vi "InitCam3001.vi"(7 "error in (no error)":errorcluster, 8 "trigger_input":u16, 10 "IS_AREA":u16) -> (0 "error out":errorcluster)   [LabVIEW 2015, in "ESLSCDLL.lvlib"]
uses:
  ESLSCDLL.lvlib
  Globals.vi
  ESLSCDLL.dll
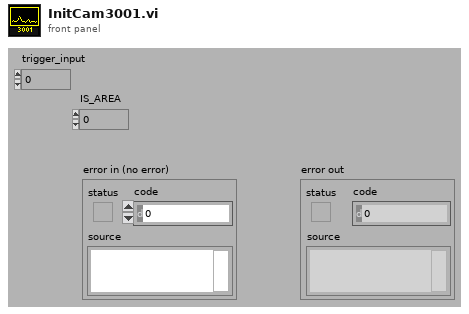
[diagram p1: front panel]
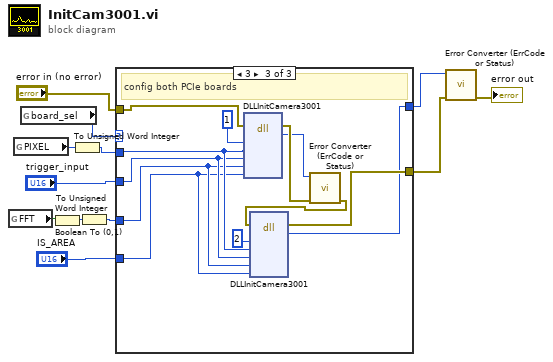
[diagram p0: block diagram]
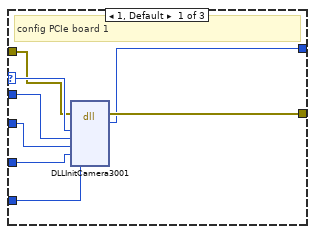
[diagram p2: hidden frame]
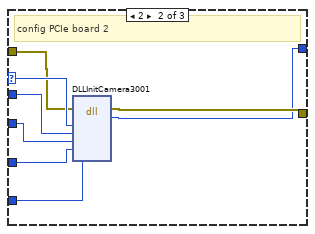
[diagram p3: hidden frame]
diagram:
  n1 = global read "Globals.vi" "FFT"() -> (w5:bool)
  n2 = global read "Globals.vi" "PIXEL"() -> (w2:u32)
  n3 = global read "Globals.vi" "board_sel"() -> (w6:u32)
  n4 = Boolean To (0,1)(Boolean=w5) -> (0, 1=w4:i16)
  n5 = To Unsigned Word Integer(number=w2) -> (unsigned 16bit integer=w1:u16)
  n6 = To Unsigned Word Integer(number=w4) -> (unsigned 16bit integer=w3:u16)
  n7 = case shown="3" w6 {
    selector: w6 -> [w20 w28 _]
    tunnel: w1 -> [w19 w27 w38]
    tunnel: "trigger_input" -> [w18 w26 w37]
    tunnel: w3 -> [w17 w25 w36]
    tunnel: "IS_AREA" -> [w16 w24 w35]
    tunnel: "error in (no error)" -> [w15 w23 w34]
    tunnel: [w14 w22 w30] -> w8
    tunnel: [w13 w21 w29] -> w7
    frame 1, Default {
      # "config PCIe board 1"
      n8 = dll-call lib="C:/Users/flori/Nextcloud/Dokumente/Stresing/Windows/lv64/board.vis/ESLSCDLL.dll" fn="DLLInitCamera3001" ("lwlscdll.dll:DLLWriteLongS0")(error in=w15, "drvno"=w20, "pixel"=w19, "trigger_input"=w18, "IS_FFT"=w17, "IS_AREA"=w16) -> (error out=w14:errorcluster, "es_status_codes"=w13:i32)  [unwired: 7 in, 1 out]
    }
    frame 2 {
      # "config PCIe board 2"
      n9 = dll-call lib="C:/Users/flori/Nextcloud/Dokumente/Stresing/Windows/lv64/board.vis/ESLSCDLL.dll" fn="DLLInitCamera3001" ("lwlscdll.dll:DLLWriteLongS0")(error in=w23, "drvno"=w28, "pixel"=w27, "trigger_input"=w26, "IS_FFT"=w25, "IS_AREA"=w24) -> (error out=w22:errorcluster, "es_status_codes"=w21:i32)  [unwired: 7 in, 1 out]
    }
    frame 3 {
      # "config both PCIe boards"
      n10 = dll-call lib="C:/Users/flori/Nextcloud/Dokumente/Stresing/Windows/lv64/board.vis/ESLSCDLL.dll" fn="DLLInitCamera3001" ("lwlscdll.dll:DLLWriteLongS0")(error in=w34, "drvno"=u32 1, "pixel"=w38, "trigger_input"=w37, "IS_FFT"=w36, "IS_AREA"=w35) -> (error out=w33:errorcluster, "es_status_codes"=w32:i32)  [unwired: 7 in, 1 out]
      n11 = call "Error Converter (ErrCode or Status).vi"("error in (no error)"=w33, "error code"=w32) -> ("error out"=w31:errorcluster)  [unwired: 9 in]
      n12 = dll-call lib="C:/Users/flori/Nextcloud/Dokumente/Stresing/Windows/lv64/board.vis/ESLSCDLL.dll" fn="DLLInitCamera3001" ("lwlscdll.dll:DLLWriteLongS0")(error in=w31, "drvno"=u32 2, "pixel"=w38, "trigger_input"=w37, "IS_FFT"=w36, "IS_AREA"=w35) -> (error out=w30:errorcluster, "es_status_codes"=w29:i32)  [unwired: 7 in, 1 out]
    }
  }
  n13 = call "Error Converter (ErrCode or Status).vi"("error in (no error)"=w8, "error code"=w7) -> ("error out"=→"error out":errorcluster)  [unwired: 9 in]
